vi "LoadOffsets.vi"(8 "error in (no error)":errorcluster) -> (0 "error out":errorcluster)   [LabVIEW 2014]
uses:
  <vilib>/Utility/config.llb/Read Key (Double).vi
  Robot Global Data.vi
  <vilib>/Utility/config.llb/NI_LVConfig.lvlib
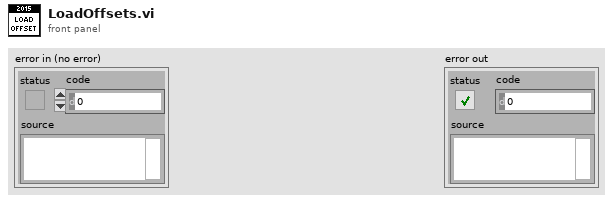
[diagram p1: front panel]
types:
  T1 = typedef "NI_LVConfig.lvlib/Config Data RefNum.ctl" = refnum<k1>
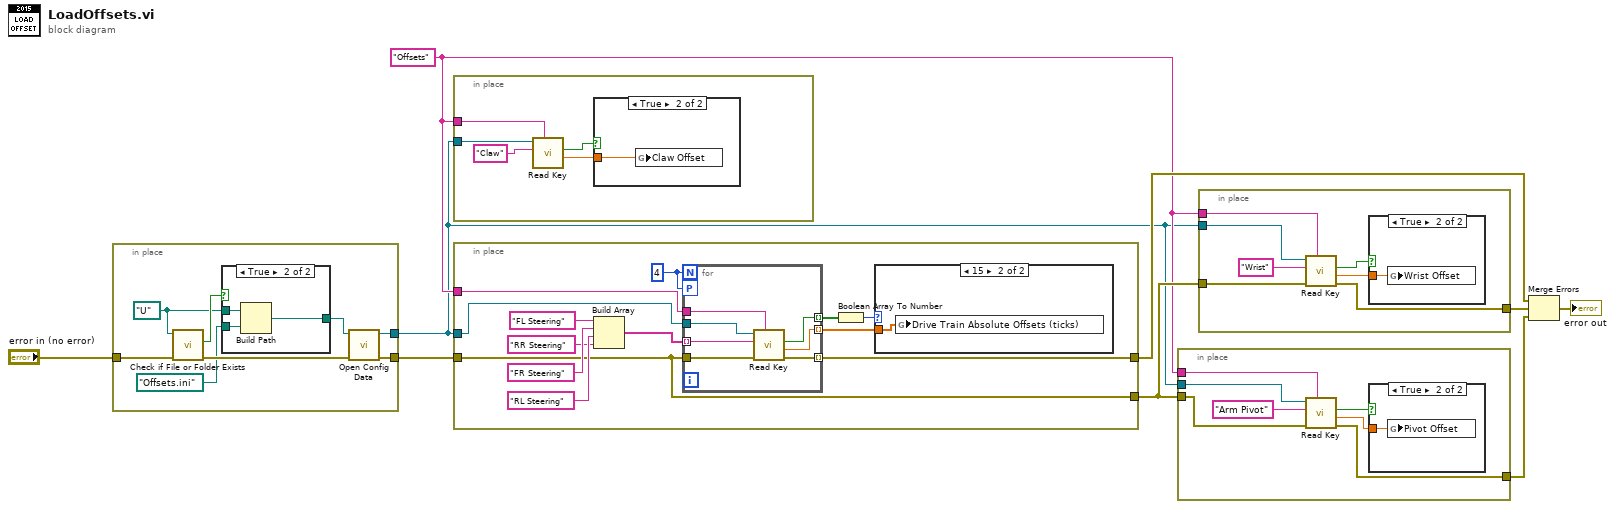
[diagram p0: block diagram]
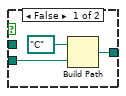
[diagram p2: hidden frame]
diagram:
  w3 = "Offsets" ("section")
  n1 = in-place {
    in-place-border: "error in (no error)" -> [w17]
    in-place-border: [w15] -> w2
    in-place-border: [w14] -> w1
    w10 = path "U:/" ("base path")
    n2 = call <vilib>:"Check if File or Folder Exists.vi"("error in (no error)"=w17, "path"=w10) -> ("error out"=w16:errorcluster, "file or folder exists?"=w11:bool)  [unwired: 7 in, 1 out]
    n3 = case shown="True" w11 {
      tunnel: path "Offsets.ini" ("default name") -> [w20 w21]
      tunnel: [w19 w22] -> w13
      tunnel: w10 -> [_ w23]
      frame False {
        n4 = Build Path(base path=path "C:/", name or relative path=w20) -> (appended path=w19:path)
      }
      frame True {
        n5 = Build Path(base path=w23, name or relative path=w21) -> (appended path=w22:path)
      }
    }
    n6 = call <vilib>:"Open Config Data.vi"("error in (no error)"=w16, "configuration file path"=w13) -> ("error out"=w15:errorcluster, "refnum"=w14:T1)  [unwired: 1 in, 7 out]
  }
  n7 = in-place {
    in-place-border: w3 -> [w28]
    in-place-border: w1 -> [w27]
    n8 = call-poly <vilib>:"Read Key.vi"("section"=w28, "key"="Claw", "refnum"=w27) -> ("value"=w24:dbl, "found?"=w25:bool)  [unwired: 5 in, 2 out]
    n9 = case shown="True" w25 {
      tunnel: w24 -> [_ w29]
      frame False {
      }
      frame True {
        n10 = global write "Robot Global Data.vi" "Claw Offset"(w29) -> ()
      }
    }
  }
  n11 = in-place {
    in-place-border: w2 -> [w31]
    in-place-border: [w36] -> w8
    in-place-border: [w31] -> w5
    in-place-border: w3 -> [w34]
    in-place-border: w1 -> [w30]
    w42 = 4
    n12 = Build Array("FL Steering", "FR Steering" ("element"), "RL Steering" ("element"), "RR Steering" ("element")) -> (w37:string[])
    n13 = for {
      N: w42 -> [_]
      workers-P: w42 -> [_]
      tunnel: w37 -> [w50] mode=indexing
      tunnel: w30 -> [w49]
      tunnel: [w48] -> w35 mode=indexing
      tunnel: w31 -> [w47]
      tunnel: [w46] -> w36 mode=indexing
      tunnel: w34 -> [w45]
      tunnel: [w44] -> w33 mode=indexing
      n14 = call-poly <vilib>:"Read Key.vi"("section"=w45, "error in (no error)"=w47, "key"=w50, "refnum"=w49) -> ("error out"=w46:errorcluster, "value"=w48:dbl, "found?"=w44:bool)  [unwired: 4 in, 1 out]
    }
    n15 = Boolean Array To Number(Boolean array=w33) -> (number=w32:u32)
    n16 = case shown="15" w32 {
      tunnel: w35 -> [_ w43]
      frame Default {
      }
      frame 15 {
        n17 = global write "Robot Global Data.vi" "Drive Train Absolute Offsets (ticks)"(w43) -> ()
      }
    }
  }
  n18 = in-place {
    in-place-border: w5 -> [w57]
    in-place-border: [w56] -> w4
    in-place-border: w3 -> [w53]
    in-place-border: w1 -> [w52]
    n19 = call-poly <vilib>:"Read Key.vi"("section"=w53, "error in (no error)"=w57, "key"="Arm Pivot", "refnum"=w52) -> ("error out"=w56:errorcluster, "value"=w54:dbl, "found?"=w51:bool)  [unwired: 4 in, 1 out]
    n20 = case shown="True" w51 {
      tunnel: w54 -> [_ w58]
      frame False {
      }
      frame True {
        n21 = global write "Robot Global Data.vi" "Pivot Offset"(w58) -> ()
      }
    }
  }
  n22 = in-place {
    in-place-border: [w65] -> w6
    in-place-border: w5 -> [w64]
    in-place-border: w3 -> [w61]
    in-place-border: w1 -> [w60]
    n23 = call-poly <vilib>:"Read Key.vi"("section"=w61, "error in (no error)"=w64, "key"="Wrist", "refnum"=w60) -> ("error out"=w65:errorcluster, "value"=w62:dbl, "found?"=w59:bool)  [unwired: 4 in, 1 out]
    n24 = case shown="True" w59 {
      tunnel: w62 -> [_ w66]
      frame False {
      }
      frame True {
        n25 = global write "Robot Global Data.vi" "Wrist Offset"(w66) -> ()
      }
    }
  }
  n26 = Merge Errors(w8, w6, w4) -> (→"error out":errorcluster)
